vi "Main SimulationV2.vi"() -> ()   [LabVIEW 2020]
panel:
  in  "Plot value\nchanges?":bool
  in  "Terminate \nProgram":bool
  out "Rf for Max i;  R+ C (EDL+Funct)":dbl
  out "Rf for Max i;  R+ C (EDL+Funct+ Analyte)":dbl
  in  "Max V_out":dbl
  out "Delta i":dbl
  out "Max i;  R+ C (EDL+Funct+ Analyte)":dbl format="%#_9e"
  out "Max i;  R+ C (EDL+Funct)":dbl format="%#_9e"
  out "V_Zeta":dbl
  out "|Z| of R+ C (EDL+Funct+Analyte)":dbl
  out "|Z| of R+ C (EDL+Funct)":dbl
  out "Delta Total Impedance":dbl
  out "Total Impedance Rs+C(EDS+Funct+Analyte)":dbl
  out "Total Impedance Rs+C(EDS+Funct)":dbl
  in  "Series Resistance of Solution":dbl
  in  "Freq Hz-MHz":dbl
  out "Impedance of EDL & Functionalization & Analyte":dbl
  out "Impedance of EDL & Functionalization":dbl
  in  "Frequency":dbl
  out "Delta C":dbl
  out "Capacitance of ELD & Functionalization & Analyte":dbl
  out "Capacitance of ELD & Functionalization":dbl
  out "C_EDL/ 1 NS":dbl
  out "C_EDL/ 1 CNT":dbl
  out "C EDL by d with Cosh Factor":dbl format="%#_6e"
  out "C EDL by d":dbl
  out "d; EDL Length":dbl
  out "R=kN_a":dbl
  out "F=eN_a":dbl
  out "N_a; Avagadro no":dbl=1.38064852e-23
  in  "V  nV-m V-V":dbl
  out "C_EDL/ A":dbl format="%#_6e"
  out "c; Charge on e":dbl=1.6021766208e-19
  in  "V zeta":dbl
  out "C in M":dbl
  in  "Co nM-M":dbl
  in  "T":dbl
  out "k; Boltzmann Constant":dbl=1.38064852e-23
  in  "Co; miliMolar (moles/m3)":dbl
  in  "er":dbl
  out "eo; Permitivity of Free Space":dbl=8.85418782e-12
  in  "z":dbl
  out "Length of CNTs  2":dbl
  in  "Dielectric of Molecule 2 Analyte":dbl
  out "Capacitance Functinal Analyte  per unit area":dbl
  out "Capaciatance per CNT Analyte":dbl
  out "Capacitance Functional Analyte per NS":dbl
  out "Capacitance Functional Analyte per NS 2":dbl
  out "Gap B/w NS":dbl
  out "Chip Impedance":dbl
  out "Chip Capacitance":dbl
  out "Chip Energy":dbl
  out "Chip Power":dbl
  in  "Freq Hz K; M Hz":dbl
  out "Power":dbl
  in  "Frequency":dbl
  out "Impedance":dbl
  in  "Voltage":dbl
  out "Energy":dbl
  out "Capacitance of 1 Pair NS":dbl(graph)
  out "Capacitance of 1 Pair NS":dbl
  in  "er":dbl
  out "Capacitance Functional Molecules per NS 2":dbl
  out "Capacitance Functional Molecules per NS":dbl
  out "Capaciatance per CNT Functional":dbl
  out "Capacitance Functinal Molecule  per unit area":dbl
  in  "Dielectric of Molecule":dbl
  out "Concentration,  M":ext[unit]
  out "Concentration on 1 NS (Moles/m3)":ext[unit]
  out "Total Functionalized Molecules on NS":dbl
  out "No of Molecules on 1 CNT Functionalized":dbl
  out "Molecule Length Analyte":dbl
  out "Molecle Area with Gap Analyte":dbl
  out "Volume of Molecule Analyte":dbl
  out "Area of Molecule on CNT surface Analyte":dbl
  in  "m-nm Gap Molecules Analyte":dbl caption="m-nm Gap"
  in  "Gap Between Molecules Analyte":dbl caption="Gap Between CNTs"
  in  "m-nm l Molecule Analyte":dbl
  in  "m-nm r Molecule Analyte":dbl caption="m-nm r"
  in  "Length of Molecule Analyte":dbl caption="Length of CNTs"
  in  "Radius of Molecule Analyte":dbl caption="Radius of CNTs"
  out "Molecule Length":dbl
  out "Molecle Area with Gap":dbl
  out "Volume of Molecule":dbl
  out "Area of Molecule on CNT surface":dbl
  in  "m-nm Gap Molecules":dbl caption="m-nm Gap"
  in  "Gap Between Molecules":dbl caption="Gap Between CNTs"
  in  "m-nm l Molecule":dbl
  in  "m-nm r Molecule":dbl caption="m-nm r"
  in  "Length of Molecule":dbl caption="Length of CNTs"
  in  "Radius of Molecule":dbl caption="Radius of CNTs"
  out "NS Width":dbl
  out "No of NS Pairs on Chip":dbl
  in  "Gap n-m":dbl
  in  "Gap B/W NS":dbl
  in  "m-nm LChip":dbl
  in  "m-nm WChip":dbl
  in  "Length of Chip":dbl
  in  "Width of Chip":dbl
  out "Surface Area 1 NS":dbl
  out "# of CNTs in 1 NS":dbl format="%#_6e"
  out "Area 1 CNT & Gap":dbl
  out "NS Length":dbl
  out "NS Base Area":dbl
  out "CNT Radius":dbl
  out "CNT Base Area":dbl
  out "XY Graph":cluster{"X":dbl[], "Y":dbl[]}[](graph)
  in  "m-nm NS Base":dbl caption="m-nm 4"
  in  "m-nm WB":dbl
  in  "Length of Base":dbl
  in  "Width of Base":dbl
  in  "m-nm Gap":dbl
  in  "Gap Between CNTs":dbl
  out "Surface Area of 1 CNT":dbl
  in  "m-nm l":dbl
  in  "m-nm r":dbl
  in  "Length of CNTs":dbl
  in  "Radius of CNTs":dbl
  # "CAP"
  # "Chip CAP"
  # "Chip NanoStructure"
  # "CNT Nanostructure"
  # "Nano Structure"
  # "Chip"
  # "Control Center"
  # "Analyte Molecule"
  # "Functionalization Molecule"
  # "Analyte Attached to Functionalized  NanoStructure"
  # "Capacitance of Analyte Molecule on NanoStructure"
  # "Functionalized NanoStructure"
  # "Molecule Fnctionalization"
  # "Capacitance of Functional Molecule on NanoStructure"
  # "Echem & Electrical Signals"
  # "Electric Double Layer; EDL"
  # "Constants"
  # "Cosh(zeV_zeta/2kT)"
  # "Potentiostat"
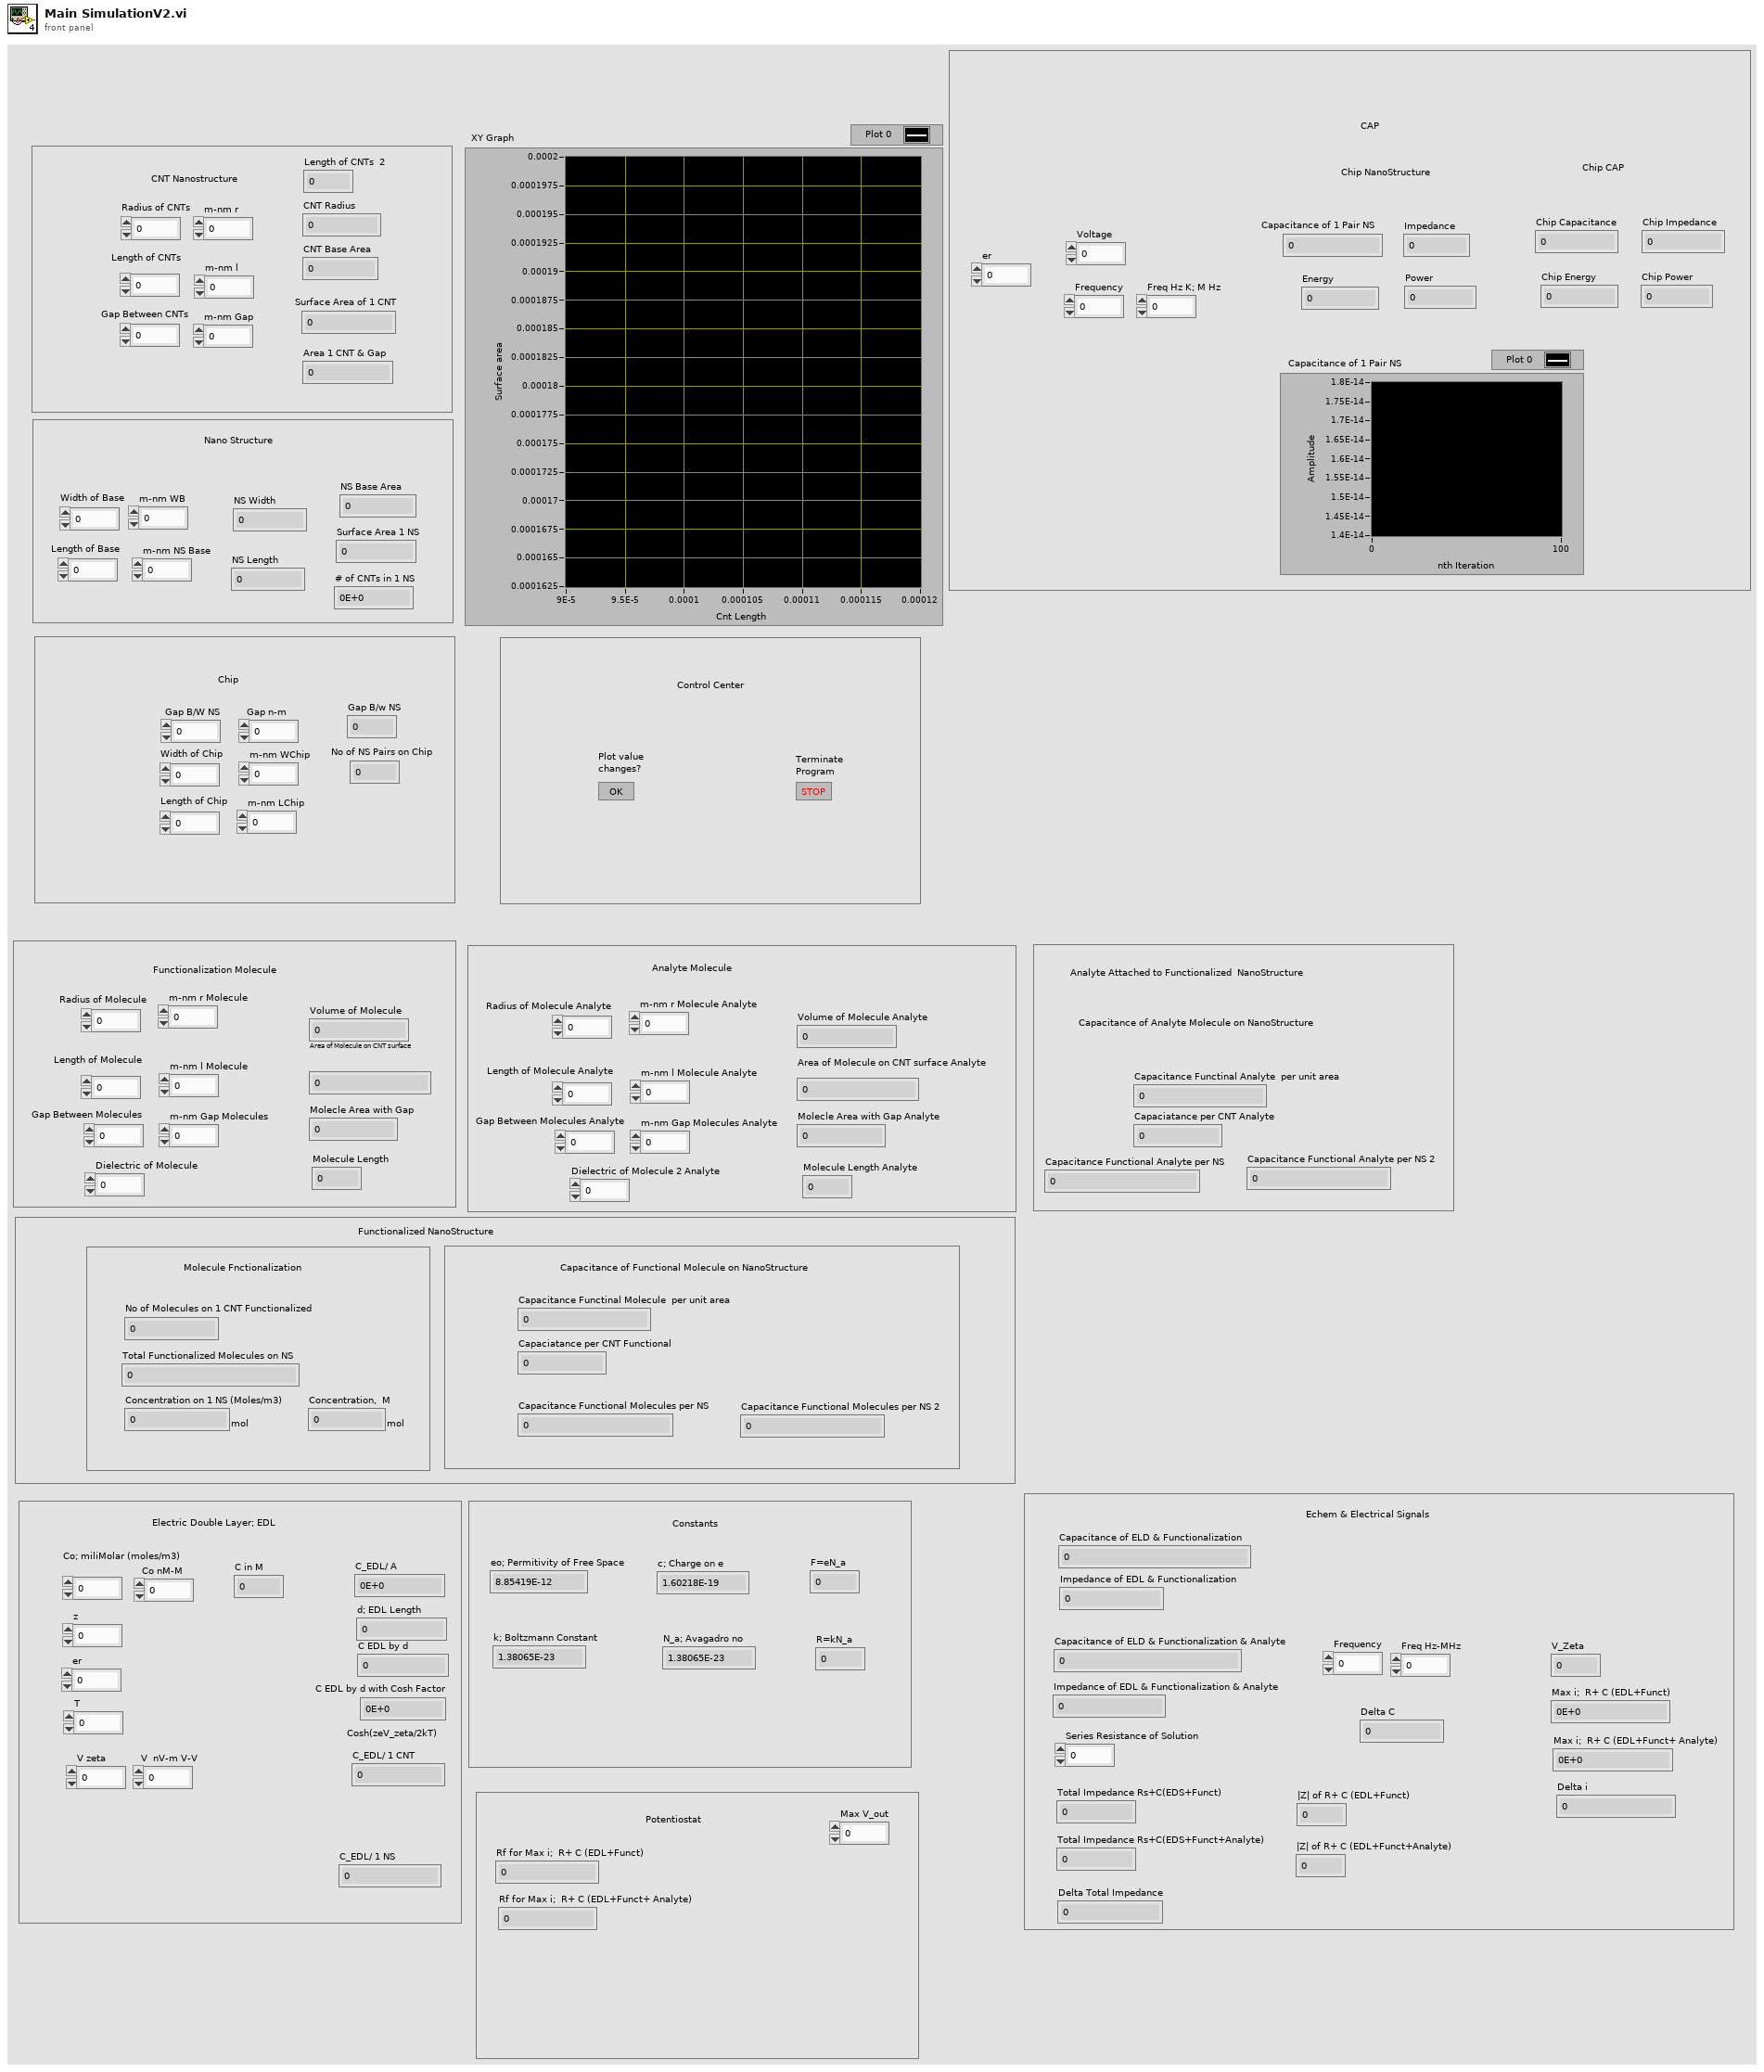
[diagram p1: front panel]
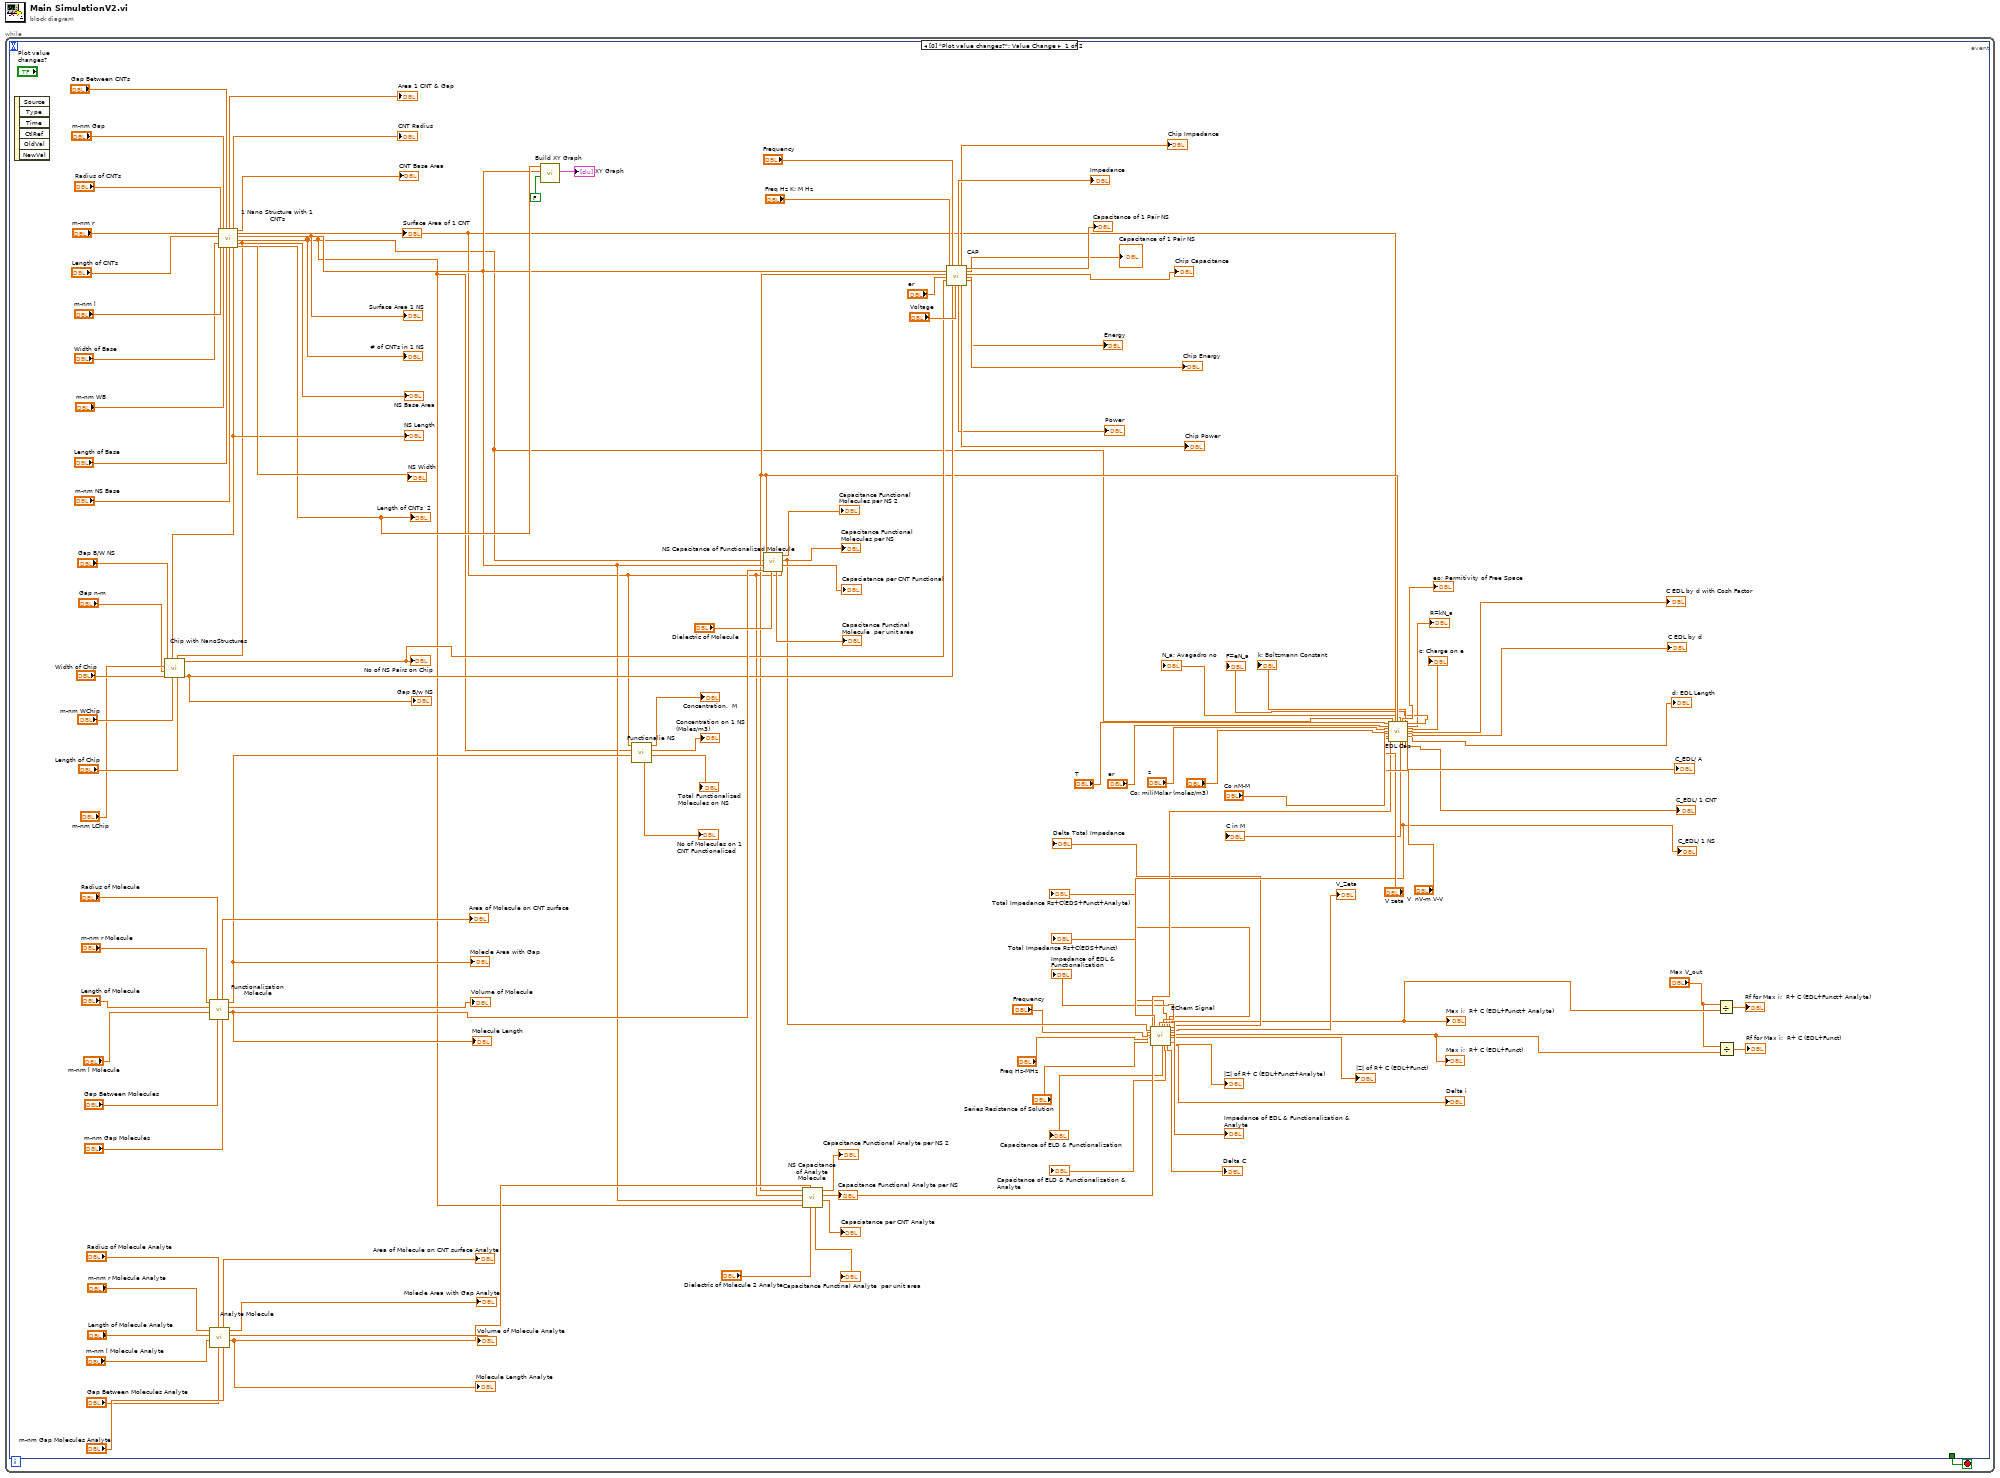
[diagram p0: block diagram]
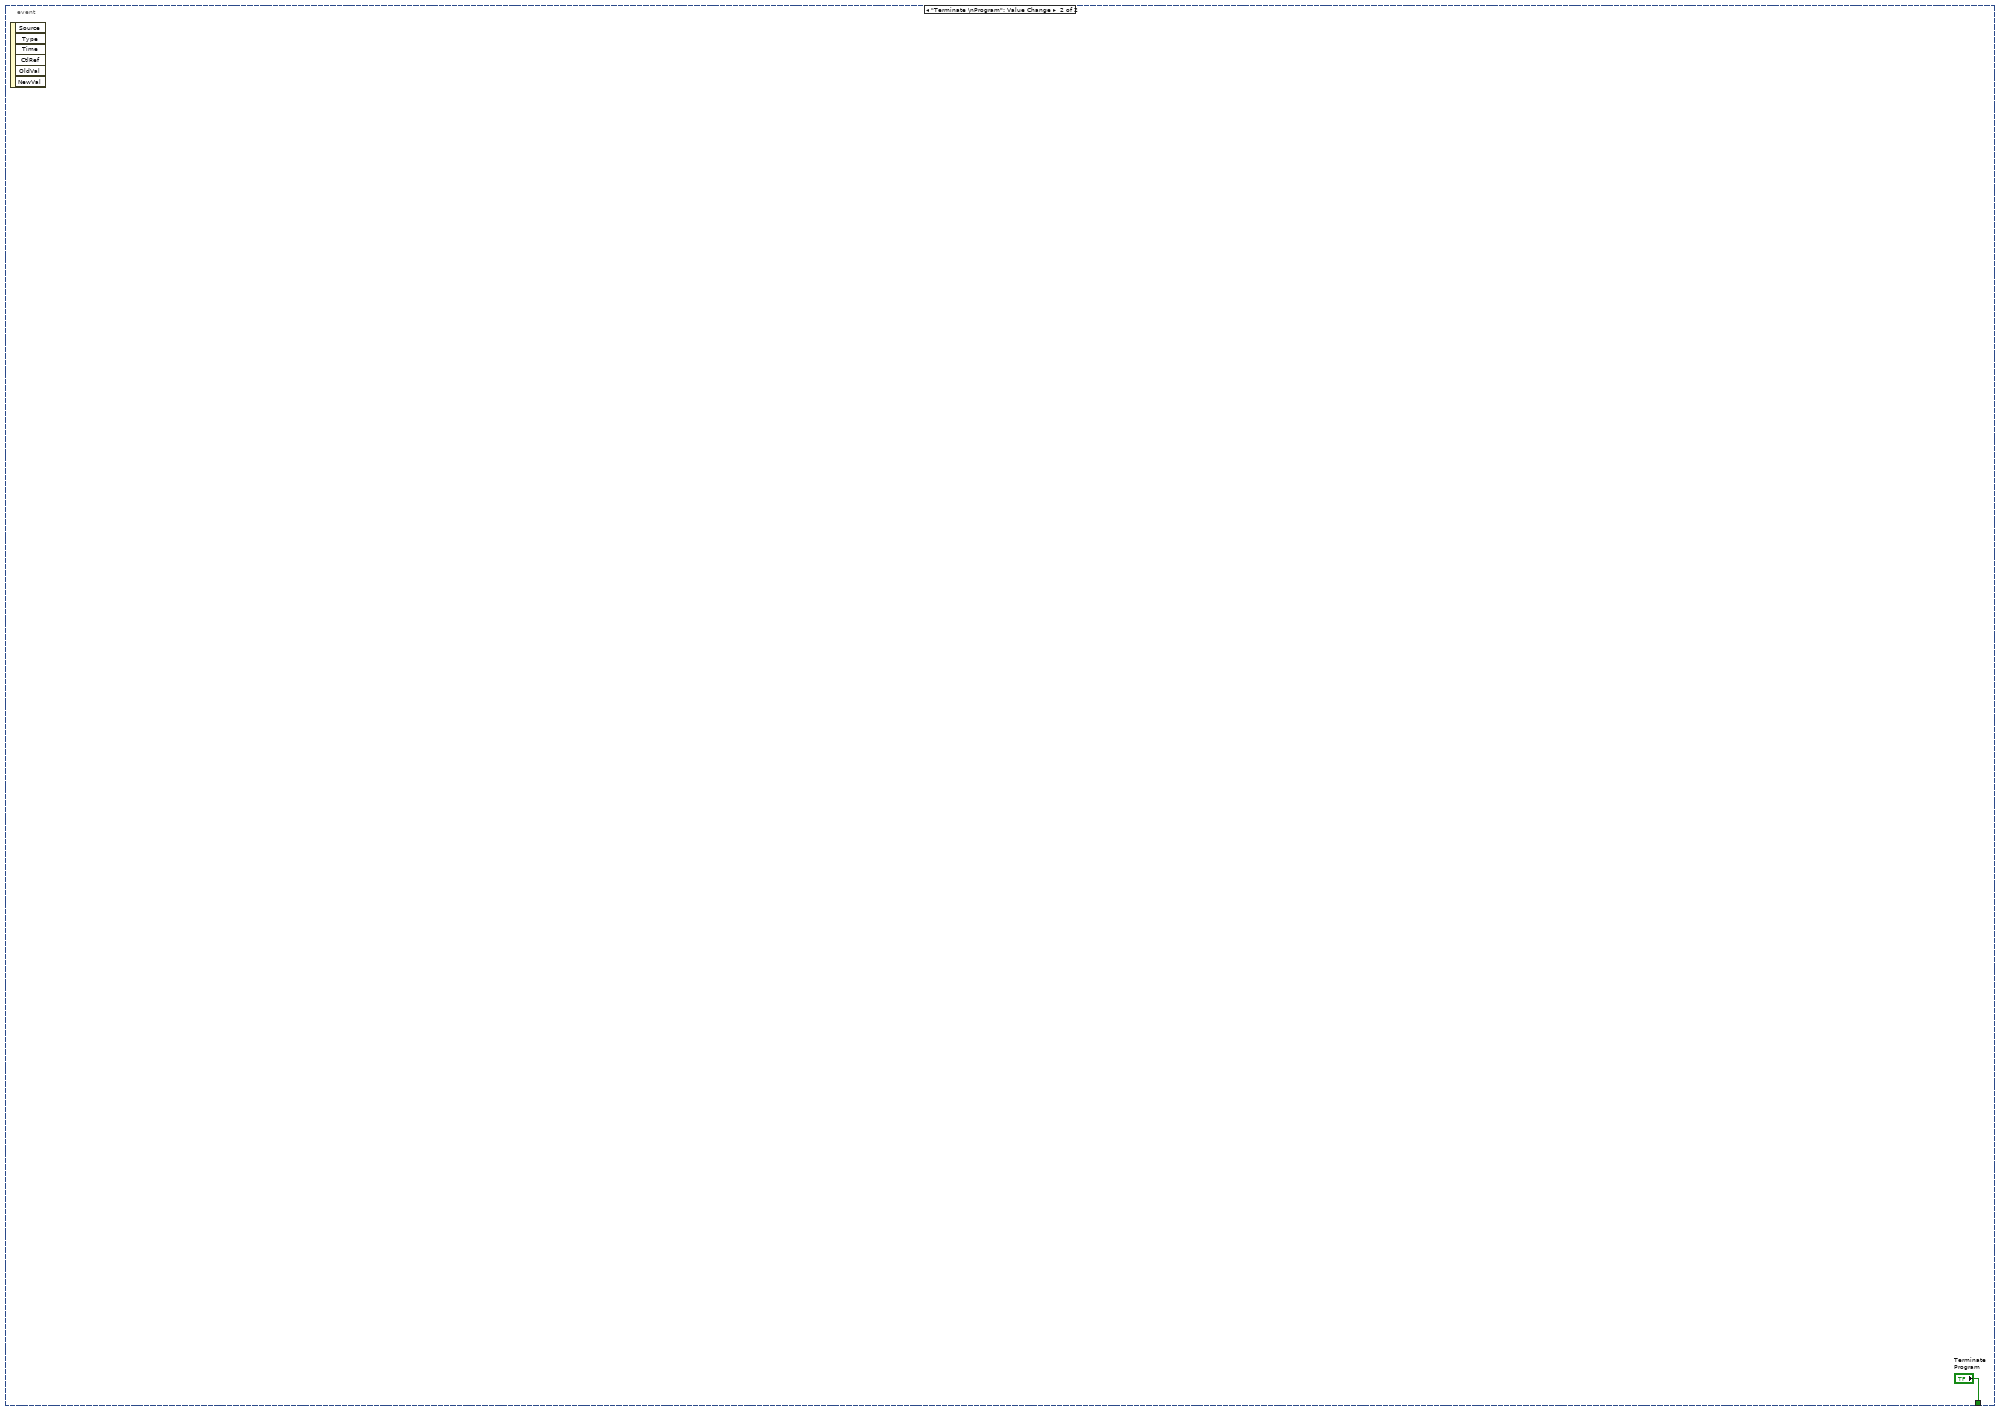
[diagram p2: hidden frame]
diagram:
  n1 = while {
    stop <- w1 stop-if-true
    n2 = event shown="[0] \"Plot value changes?\": Value Change" {
      selector: _ -> [_ _]
      dyn-events: _ -> [_ _]
      timeout: _ -> [_ _]
      tunnel: [_ "Terminate \nProgram"] -> w1
      event "Plot value\nchanges?": Value Change {
        n3 = event-data() -> ()  [unwired: 1 in, 6 out]
        n4 = call "Functionalization Molecule.vi"("m-nm Gap Molecules"="m-nm Gap Molecules", "Gap Between Molecules"="Gap Between Molecules", "Radius of Molecule"="Radius of Molecule", "m-nm l Molecule"="m-nm l Molecule", "Length of Molecule"="Length of Molecule", "m-nm r Molecule"="m-nm r Molecule") -> ("Molecule Length"=w78:dbl, "Volume of Molecule"=→"Volume of Molecule":dbl, "Molecle Area with Gap"=w84:dbl, "Area of Molecule on CNT surface"=→"Area of Molecule on CNT surface":dbl)  [unwired: 2 in]
        "Molecle Area with Gap" <- w84
        "Molecule Length" <- w78
        n5 = call "Analyte Molecule.vi"("m-nm Gap Molecules"="m-nm Gap Molecules Analyte", "Gap Between Molecules"="Gap Between Molecules Analyte", "Radius of Molecule"="Radius of Molecule Analyte", "m-nm l Molecule"="m-nm l Molecule Analyte", "Length of Molecule"="Length of Molecule Analyte", "m-nm r Molecule"="m-nm r Molecule Analyte") -> ("Molecule Length"=w57:dbl, "Volume of Molecule"=→"Volume of Molecule Analyte":dbl, "Molecle Area with Gap"=→"Molecle Area with Gap Analyte":dbl, "Area of Molecule on CNT surface"=→"Area of Molecule on CNT surface Analyte":dbl)  [unwired: 2 in]
        "Molecule Length Analyte" <- w57
        n6 = call "1 Nano Structure with 1 CNTs.vi"("Radius of CNTs"="Radius of CNTs", "m-nm r"="m-nm r", "Length of CNTs"="Length of CNTs", "m-nm l"="m-nm l", "Width of Base"="Width of Base", "m-nm Gap"="m-nm Gap", "m-nm WB"="m-nm WB", "Gap Between CNTs"="Gap Between CNTs", "Length of Base"="Length of Base", "m-nm NS Base"="m-nm NS Base") -> ("Length of CNTs"=w54:dbl, "Area 1 CNT & Gap"=→"Area 1 CNT & Gap":dbl, "CNT Radius"=→"CNT Radius":dbl, "NS Length"=w100:dbl, "CNT Base Area"=→"CNT Base Area":dbl, "Surface Area of 1 CNT"=w44:dbl, "Surface Area 1 NS"=w53:dbl, "# of CNTs in 1 NS"=w43:dbl, "NS Base Area"=w99:dbl, "NS Width"=→"NS Width":dbl)
        "Surface Area of 1 CNT" <- w44
        "NS Base Area" <- w99
        "NS Length" <- w100
        "# of CNTs in 1 NS" <- w43
        "Surface Area 1 NS" <- w53
        "Length of CNTs  2" <- w54
        n7 = call "Chip with NanoStructures.vi"("Length of Chip"="Length of Chip", "NS Base Area"=w99, "m-nm WChip"="m-nm WChip", "NS Length"=w100, "Width of Chip"="Width of Chip", "Gap n-m"="Gap n-m", "m-nm LChip"="m-nm LChip", "Gap B/W NS"="Gap B/W NS") -> ("Gap B/w NS"=w70:dbl, "No of NS Pairs on Chip"=w69:dbl)  [unwired: 2 in]
        "No of NS Pairs on Chip" <- w69
        "Gap B/w NS" <- w70
        n8 = call "Build XY Graph"("Reset"=FALSE, "Y Input"=w53, "X Input"=w54) -> ("XY Graph"=→"XY Graph":cluster{"X":dbl[], "Y":dbl[]}[])  [unwired: 7 in, 1 out]
        n9 = call "Functionalie NS.vi"("Molecle Area with Gap"=w84, "# of CNTs in 1 NS"=w43, "Surface Area of 1 CNT"=w44) -> ("Total Functionalized Molecules on NS"=→"Total Functionalized Molecules on NS":dbl, "Concentration on 1 NS (Moles/m3)"=→"Concentration on 1 NS (Moles/m3)":ext[unit], "Concentration,  M"=→"Concentration,  M":ext[unit], "No of Molecules on 1 CNT Functionalized"=→"No of Molecules on 1 CNT Functionalized":dbl)  [unwired: 5 in]
        n10 = call "EDL Cap.vi"("T"="T", "er"="er", "z"="z", "Co; miliMolar (moles/m3)"="Co; miliMolar (moles/m3)", "Co nM-M"="Co nM-M", "V  nV-m V-V"="V  nV-m V-V", "V zeta"="V zeta", "# of CNTs in 1 NS"=w43, "Surface Area of 1 CNT"=w44) -> ("V_Zeta"=w23:dbl, "eo; Permitivity of Free Space 2"=w45:dbl, "N_a; Avagadro no"=→"N_a; Avagadro no":dbl, "C in M"=→"C in M":dbl, "eo; Permitivity of Free Space"=→"eo; Permitivity of Free Space":dbl, "C_EDL/ 1 NS"=w28:dbl, "k; Boltzmann Constant"=→"k; Boltzmann Constant":dbl, "C_EDL/ 1 CNT"=→"C_EDL/ 1 CNT":dbl, "F=eN_a"=→"F=eN_a":dbl, "R=kN_a"=→"R=kN_a":dbl, "c; Charge on e"=→"c; Charge on e":dbl, "C EDL by d with Cosh Factor"=→"C EDL by d with Cosh Factor":dbl, "C EDL by d"=→"C EDL by d":dbl, "d; EDL Length"=→"d; EDL Length":dbl, "C_EDL/ A"=→"C_EDL/ A":dbl)  [unwired: 4 in]
        "C_EDL/ 1 NS" <- w28
        n11 = call "NS Capacitance of Functionalized Molecule.vi"("SA of 1 CNT"=w44, "Dielectric of Molecule"="Dielectric of Molecule", "Molecule Length"=w78, "Surface Area 1 NS"=w53, "# of CNTs"=w43, "Permitivity of Free Space"=w45) -> ("Capaciatance per CNT"=→"Capaciatance per CNT Functional":dbl, "Capacitance Functional Molecules per NS"=w29:dbl, "Capacitance Functional Molecules per NS 2"=→"Capacitance Functional Molecules per NS 2":dbl, "Capacitance Functinal Molecule  per unit area"=→"Capacitance Functinal Molecule  per unit area":dbl)  [unwired: 2 in]
        "Capacitance Functional Molecules per NS" <- w29
        n12 = call "NS Capacitance of Analyte Molecule.vi"("Dielectric of Molecule Analyte"="Dielectric of Molecule 2 Analyte", "Molecule Length"=w57, "# of CNTs"=w43, "Surface Area 1 NS"=w53, "Surface Area of 1 CNT"=w44, "Permitivity of Free Space"=w45) -> ("Capaciatance per CNT"=→"Capaciatance per CNT Analyte":dbl, "Capacitance Functional Analyte per NS"=w30:dbl, "Capacitance Functional Analyte per NS 2"=→"Capacitance Functional Analyte per NS 2":dbl, "Capacitance Functinal Analyte  per unit area"=→"Capacitance Functinal Analyte  per unit area":dbl)  [unwired: 2 in]
        "Capacitance Functional Analyte per NS" <- w30
        n13 = call "CAP.vi"("Freq Hz K; M Hz"="Freq Hz K; M Hz", "Surface Area 1 NS"=w53, "Permitivity of Free Space"=w45, "er"="er", "No of NS Pairs on Chip"=w69, "Frequency"="Frequency", "Gap B/w NS"=w70, "Voltage"="Voltage") -> ("Impedance"=→"Impedance":dbl, "Power"=→"Power":dbl, "Chip Impedance"=→"Chip Impedance":dbl, "Chip Power"=→"Chip Power":dbl, "Capacitance of 1 Pair NS"=→"Capacitance of 1 Pair NS":dbl, "Capacitance of 1 Pair"=→"Capacitance of 1 Pair NS":dbl, "Chip Capacitance"=→"Chip Capacitance":dbl, "Chip Energy"=→"Chip Energy":dbl, "Energy"=→"Energy":dbl)  [unwired: 3 in]
        n14 = call "EChem Signal.vi"("V_Zeta in"=w23, "Capacitance Functional Molecules per NS"=w29, "Series Resistance of Solution"="Series Resistance of Solution", "Frequency"="Frequency", "Freq Hz-MHz"="Freq Hz-MHz", "Capacitance Functional Analyte per NS"=w30, "C_EDL/ 1 NS"=w28) -> ("Impedance of EDL & Functionalization & Analyte"=→"Impedance of EDL & Functionalization & Analyte":dbl, "Impedance of EDL & Functionalization"=→"Impedance of EDL & Functionalization":dbl, "Capacitance of ELD & Functionalization"=→"Capacitance of ELD & Functionalization":dbl, "Total Impedance Rs+C(EDS+Funct)"=→"Total Impedance Rs+C(EDS+Funct)":dbl, "Capacitance of ELD & Functionalization & Analyte"=→"Capacitance of ELD & Functionalization & Analyte":dbl, "Total Impedance Rs+C(EDS+Funct+Analyte)"=→"Total Impedance Rs+C(EDS+Funct+Analyte)":dbl, "Delta C"=→"Delta C":dbl, "Delta Total Impedance"=→"Delta Total Impedance":dbl, "V_Zeta out"=→"V_Zeta":dbl, "Max i;  R+ C (EDL+Funct)"=w7:dbl, "|Z| of R+ C (EDL+Funct)"=→"|Z| of R+ C (EDL+Funct)":dbl, "Delta i"=→"Delta i":dbl, "Max i;  R+ C (EDL+Funct+ Analyte)"=w11:dbl, "|Z| of R+ C (EDL+Funct+Analyte)"=→"|Z| of R+ C (EDL+Funct+Analyte)":dbl)  [unwired: 7 in]
        "Max i;  R+ C (EDL+Funct)" <- w7
        "Max i;  R+ C (EDL+Funct+ Analyte)" <- w11
        n15 = Divide(x="Max V_out", y=w11) -> (x/y=→"Rf for Max i;  R+ C (EDL+Funct+ Analyte)":dbl)
        n16 = Divide(x="Max V_out", y=w7) -> (x/y=→"Rf for Max i;  R+ C (EDL+Funct)":dbl)
      }
      event "Terminate \nProgram": Value Change {
        n17 = event-data() -> ()  [unwired: 1 in, 6 out]
      }
    }
  }
